vi "导出参数.vi"(9 "名称或相对路径":string, 10 "基路径":path, 11 "表格控件":string[][](table)) -> ()   [LabVIEW 2021]
uses:
  <vilib>/Utility/NIReport.llb/Report Type.ctl
  <vilib>/addons/_office/excel.llb/Excel Easy Table (str).vi
  <vilib>/Utility/NIReport.llb/NI_report.lvclass
  <vilib>/addons/_office/NI_ReportGenerationToolkit.lvlib
  <vilib>/Utility/NIReport.llb/NI_ReportGenerationCore.lvlib
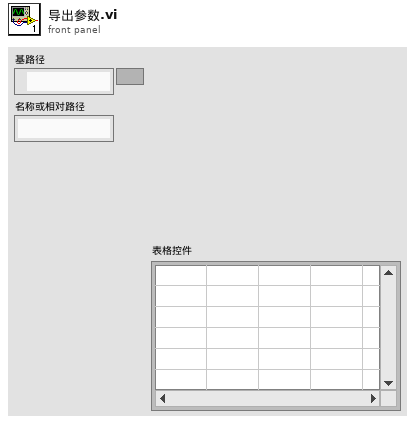
[diagram p1: front panel]
types:
  T1 = typedef "NI_ReportGenerationCore.lvlib/Report Type.ctl" = enum16{"HTML", "Word", "Excel"}
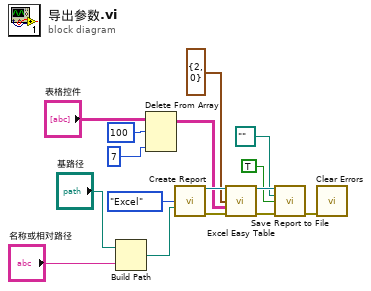
[diagram p0: block diagram]
diagram:
  n1 = Build Path(base path="基路径", name or relative path="名称或相对路径") -> (appended path=w6:path)
  n2 = Delete From Array(array="表格控件", length=100 ("长度"), index (col)=7 ("禁用的索引 (列)")) -> (array with subset deleted=w11:string[][])  [unwired: 1 in, 1 out]
  n3 = call <vilib>:"Create Report.vi"("report type"=Report_Type."Excel", "template (empty)"=w6) -> ("report out"=w16:refnum<class "NI_report.lvclass">, "error out"=w7:errorcluster)  [unwired: 12 in]
  n4 = call-poly <vilib>:"Excel Easy Table.vi"("report in"=w16, "start (0, 0)"=cluster{"row":i32, "column":i32} {"row"=2, "column"=0}, "text data"=w11, "error in (no error)"=w7) -> ("report out"=w5:refnum<class "NI_report.lvclass">, "error out"=w2:errorcluster)  [unwired: 7 in, 3 out]
  n5 = call-dynamic "Save Report to File.vi"("report in"=w5, "report file path"=path "", "prompt to replace? (F)"=TRUE, "error in (no error)"=w2) -> ("error out"=w1:errorcluster)  [unwired: 10 in, 1 out]
  n6 = call <vilib>:"Clear Errors.vi"("error in (no error)"=w1) -> ()  [unwired: 5 in, 2 out]
